vi "CLEAN.vi"(4 "Number of Strips Per Clear":u32, 5 "Number of Clears":u32, 6 "Number of Minimum blocks":u32, 7 "Minimum Block Size":u32, 8 "error out":errorcluster, 9 "Continous Clean":bool, 10 "Skip Serial Reg Clean":bool, 11 "Camera Handle":u32) -> (0 "error out 2":errorcluster, 1 "String":string, 2 "INI Flag":bool, 3 "CameraHandle":u32)   [LabVIEW 2015]
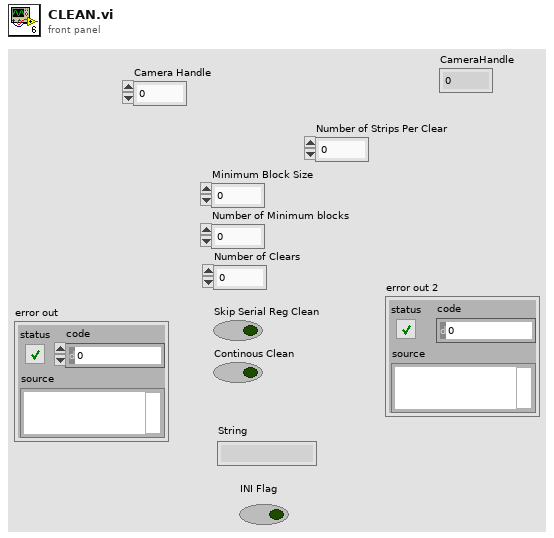
[diagram p1: front panel]
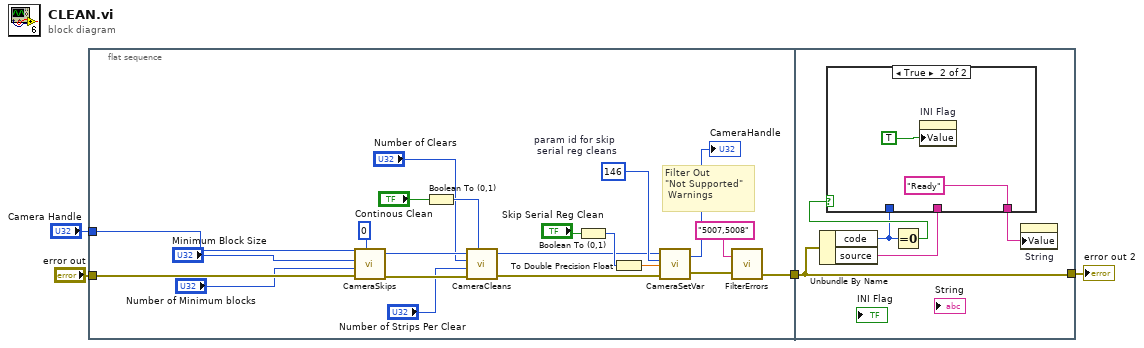
[diagram p0: block diagram]
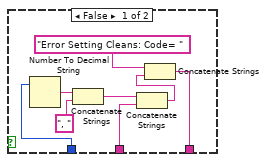
[diagram p2: hidden frame]
diagram:
  n1 = flat-sequence {
    tunnel: [w16] -> w4
    tunnel: "error out" -> [w24]
    tunnel: "Camera Handle" -> [w15]
    tunnel: w4 -> [w30]
    tunnel: [w30] -> w2
    frame #0 {
      w20 = u32 146  # param id for skip  serial reg cleans
      # "Filter Out\n\"Not Supported\"\n Warnings"
      n2 = call <userlib>:"CameraSkips.vi"("Camera Handle"=w15, "Minimum Block Size"="Minimum Block Size", "Number of Minimum blocks"="Number of Minimum blocks", "error in"=w24, "Type of Skips"=u32 0) -> ("Camera Handle"=w13:u32, "error out"=w23:errorcluster)
      n3 = Boolean To (0,1)(Boolean="Continous Clean") -> (0, 1=w10:i16)
      n4 = call <userlib>:"CameraCleans.vi"("Camera Handle"=w13, "Number of Clears"="Number of Clears", "Number of Strips Per Clear"="Number of Strips Per Clear", "error in"=w23, "Continuous Clears"=w10) -> ("Camera Handle"=w17:u32, "error out"=w18:errorcluster)
      n5 = Boolean To (0,1)(Boolean="Skip Serial Reg Clean") -> (0, 1=w21:i16)
      n6 = To Double Precision Float(number=w21) -> (double precision float=w5:dbl)
      n7 = call <userlib>:"CameraSetVar.vi"("error in"=w18, "Value"=w5, "Parameter ID"=w20, "Camera Handle"=w17) -> ("error out"=w19:errorcluster, "CameraHandle"=→"CameraHandle":u32)
      n8 = call "FilterErrors.vi"("error in (no error)"=w19, "Error Numbers To Filter"="5007,5008") -> ("error out"=w16:errorcluster)
    }
    frame #1 {
      n9 = Unbundle By Name(w30) -> ("code"=w27:i32, "source"=w28:string)
      n10 = Equal To 0?(x=w27) -> (x = 0?=w29:bool)
      n11 = case shown="True" w29 {
        tunnel: [w31 "Ready"] -> w26
        tunnel: w28 -> [w32 _]
        tunnel: w27 -> [w37 _]
        frame False {
          n12 = Number To Decimal String(number=w37) -> (decimal integer string=w36:string)  [unwired: 1 in]
          n13 = Concatenate Strings(w36, ", ") -> (w33:string)
          n14 = Concatenate Strings(w33, w32) -> (w34:string)
          n15 = Concatenate Strings("Error Setting Cleans: Code= ", w34) -> (w31:string)
        }
        frame True {
          n16 = property on="INI Flag" class="Bool (strict)"("Value"=TRUE) -> ()  [unwired: 2 in, 2 out]
        }
      }
      n17 = property on="String" class="Str"("Value"=w26) -> ()  [unwired: 2 in, 2 out]
    }
  }
  "error out 2" <- w2
